vi "Read_text_file_mic.vi"(11 "file path (dialog if empty)":path) -> (3 "Table":string[][](array[string]))   [LabVIEW 2022 SP3]
doc: "Reads a specified number of lines or rows from a numeric text file beginning at a specified character offset and converts the data to a 2D, single-precision array of numbers."
panel:
  in  "delimiter (Tab)":string="\t"
  in  "type (empty)":string[][](array[string])
  in  "format (%.3f)":string="%.3f"
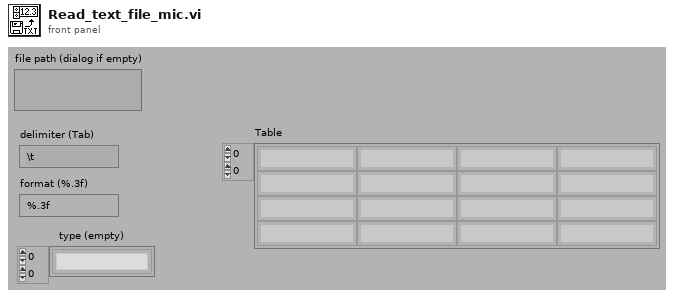
[diagram p1: front panel]
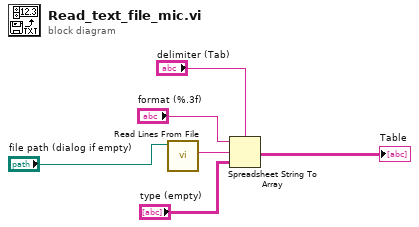
[diagram p0: block diagram]
diagram:
  n1 = call <vilib>:"Read Lines From File.vi"("file path (dialog if empty)"="file path (dialog if empty)") -> ("line string"=w5:string)  [unwired: 5 in, 3 out]
  n2 = Spreadsheet String To Array(delimiter (Tab)="delimiter (Tab)", format string="format (%.3f)", spreadsheet string=w5, array type (2D Dbl)="type (empty)") -> (array=→"Table":string[][])
